vi "Rectangle search (SubVI).vi"(10 "Minimum match score":dbl, 11 "Refnum in":T1) -> (2 "Rectangles":T2(array[cluster]) {"Corners"."Y" format="%.2f"; "Corners"."X" format="%.2f"}, 3 "Refnum out":T1)   [LabVIEW 2014]
uses:
  <vilib>/vision/Image Controls.llb/IMAQ Image.ctl
  <vilib>/vision/Shape Detection.llb/ShapeDetectionMatchOptions.ctl
  <vilib>/vision/Pattern Matching.llb/IMAQ Match Range Setting.ctl
  <vilib>/vision/Pattern Matching.llb/IMAQ Curve Parameters.ctl
  <vilib>/vision/NI_Vision_Development_Module.lvlib
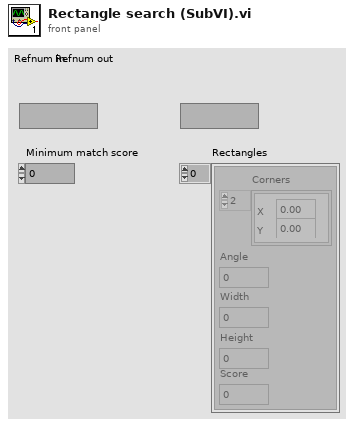
[diagram p1: front panel]
types:
  T1 = typedef "IMAQ Image.ctl" = refnum<image>
  T2 = cluster{"Corners":cluster{"X":sgl, "Y":sgl}[], "Angle":dbl, "Width":dbl, "Height":dbl, "Score":dbl}[]
  T3 = typedef "IMAQ Curve Parameters.ctl" = cluster{"Extraction Mode":u32, "Edge Threshold":i32, "Edge Filter Size":u32, "Min Length":i32, "Row Search Step Size":i32, "Col Search Step Size":i32, "Max Endpoint Gap":i32, "Closed":bool, "Subpixel":bool}
  T4 = typedef "ShapeDetectionMatchOptions.ctl" = cluster{"Rotation":bool, "Scale":bool, "Occlusion":bool, "Range Settings":T5[]}
  T5 = typedef "IMAQ Match Range Setting.ctl" = cluster{"Match Constraints":u32, "Min":dbl, "Max":dbl}
  T6 = cluster{"Min Width":dbl, "Max Width":dbl, "Min Height":dbl, "Max Height":dbl}
  T7 = cluster{"Rectangles[0]":cluster{"Corners":cluster{"X":sgl, "Y":sgl}[], "Angle":dbl, "Width":dbl, "Height":dbl, "Score":dbl}, "Rectangles[1]":cluster{"Corners":cluster{"X":sgl, "Y":sgl}[], "Angle":dbl, "Width":dbl, "Height":dbl, "Score":dbl}, "Rectangles[2]":cluster{"Corners":cluster{"X":sgl, "Y":sgl}[], "Angle":dbl, "Width":dbl, "Height":dbl, "Score":dbl}, "Rectangles[3]":cluster{"Corners":cluster{"X":sgl, "Y":sgl}[], "Angle":dbl, "Width":dbl, "Height":dbl, "Score":dbl}, "Rectangles[4]":cluster{"Corners":cluster{"X":sgl, "Y":sgl}[], "Angle":dbl, "Width":dbl, "Height":dbl, "Score":dbl}, "Rectangles[5]":cluster{"Corners":cluster{"X":sgl, "Y":sgl}[], "Angle":dbl, "Width":dbl, "Height":dbl, "Score":dbl}, "Rectangles[6]":cluster{"Corners":cluster{"X":sgl, "Y":sgl}[], "Angle":dbl, "Width":dbl, "Height":dbl, "Score":dbl}, "Rectangles[7]":cluster{"Corners":cluster{"X":sgl, "Y":sgl}[], "Angle":dbl, "Width":dbl, "Height":dbl, "Score":dbl}, "Rectangles[8]":cluster{"Corners":cluster{"X":sgl, "Y":sgl}[], "Angle":dbl, "Width":dbl, "Height":dbl, "Score":dbl}}
  T8 = cluster{"Corners":cluster{"X":sgl, "Y":sgl}[], "Angle":dbl, "Width":dbl, "Height":dbl, "Score":dbl}
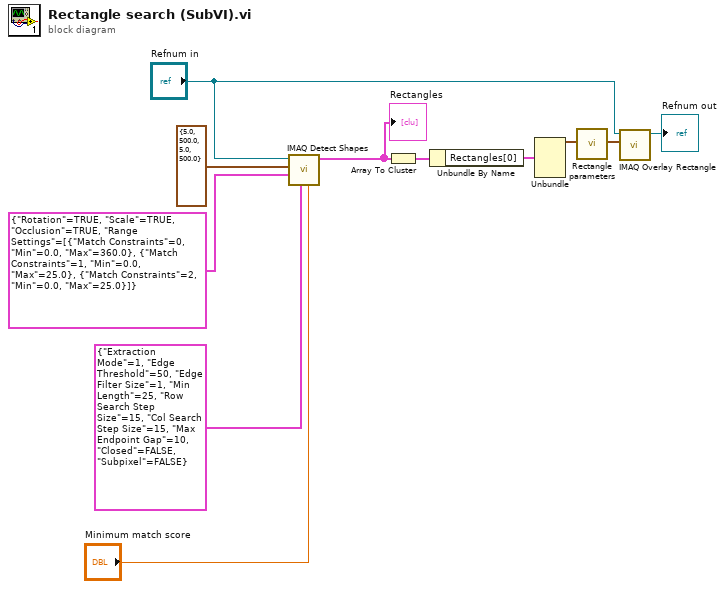
[diagram p0: block diagram]
diagram:
  n1 = call-poly "IMAQ Detect Shapes"("Minimum match score"="Minimum match score", "Curve Parameters"=T3 {"Extraction Mode"=1, "Edge Threshold"=50, "Edge Filter Size"=1, "Min Length"=25, "Row Search Step Size"=15, "Col Search Step Size"=15, "Max Endpoint Gap"=10, "Closed"=FALSE, "Subpixel"=FALSE}, "Match Options"=T4 {"Rotation"=TRUE, "Scale"=TRUE, "Occlusion"=TRUE, "Range Settings"=[{"Match Constraints"=0, "Min"=0.0, "Max"=360.0}, {"Match Constraints"=1, "Min"=0.0, "Max"=25.0}, {"Match Constraints"=2, "Min"=0.0, "Max"=25.0}]}, "Rectangle Descriptor"=T6 {"Min Width"=5.0, "Max Width"=500.0, "Min Height"=5.0, "Max Height"=500.0}, "Image"="Refnum in") -> ("Rectangles"=w4:T2)  [unwired: 4 in, 2 out]
  "Rectangles" <- w4
  n2 = Array To Cluster(array=w4) -> (cluster=w5:T7)
  n3 = Unbundle By Name(w5) -> ("Rectangles[0]"=w6:T8)
  n4 = Unbundle(w6) -> ("Corners"=w9:cluster{"X":sgl, "Y":sgl}[])  [unwired: 4 out]
  n5 = call "Rectangle parameters.vi"("Corners"=w9) -> ("Overlay Rectangle Corners"=w10:cluster{sgl, sgl, sgl, sgl})  [unwired: 18 in]
  n6 = call "IMAQ Overlay Rectangle"("Rectangle"=w10, "Image"="Refnum in") -> ("Image Out"=→"Refnum out":T1)  [unwired: 8 in, 1 out]
